vi "Is Descendant of Class.vi"(8 "error in (no error)":errorcluster, 10 "ancestor name":string, 11 "class in":refnum<vi>) -> (0 "error out":errorcluster, 2 "is descendant?":bool, 3 "class out":refnum<vi>)   [LabVIEW 2021, in "MeasurementService Editor.lvlib"]
uses:
  MeasurementService Editor.lvlib
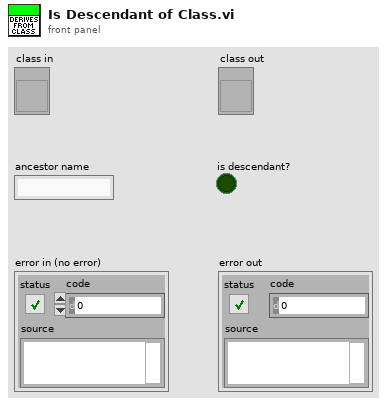
[diagram p1: front panel]
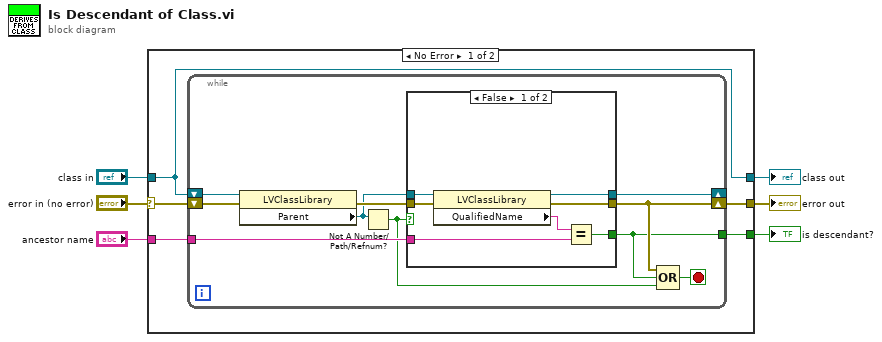
[diagram p0: block diagram]
diagram:
  n1 = case shown="No Error" "error in (no error)" {
    selector: "error in (no error)" -> [w8 w31]
    tunnel: "ancestor name" -> [w11 _]
    tunnel: "class in" -> [w7 w30]
    tunnel: [w10 w31] -> w4
    tunnel: [w9 _] -> w3
    tunnel: [w7 w30] -> w1
    frame No Error {
      n2 = while {
        shift-right: [w15] -> _
        shift-left: w7 -> [w21]
        shift-right: [w14] -> w10
        shift-left: w8 -> [w20]
        tunnel: w11 -> [w16]
        tunnel: [w13] -> w9
        stop <- w19 stop-if-true
        n3 = property class="LVClassLibrary"(reference=w21, error in=w20) -> (error out=w18:errorcluster, "Parent"=w17:refnum<vi>)  [unwired: 1 out]
        n4 = Not A Number/Path/Refnum?(number/path/refnum=w17) -> (NaN/Path/Refnum?=w12:bool)
        n5 = case shown="False" w12 {
          tunnel: w18 -> [w28 w29]
          tunnel: w17 -> [w27 _]
          tunnel: w16 -> [w26 _]
          tunnel: [w25 _] -> w13
          tunnel: [w22 w29] -> w14
          tunnel: [w24 _] -> w15
          frame False {
            n6 = property class="LVClassLibrary"(reference=w27, error in=w28) -> (reference out=w24:refnum<vi>, error out=w22:errorcluster, "QualifiedName"=w23:string)
            n7 = Equal?(x=w23, y=w26) -> (x = y?=w25:bool)
          }
          frame True {
          }
        }
        n8 = Compound Arithmetic op=OR(w14, w13, w12) -> (w19:bool)
      }
    }
    frame Error {
    }
  }
  "error out" <- w4
  "is descendant?" <- w3
  "class out" <- w1
